vi "CRC16-接收校验.vi"(0 "读取缓冲区":string) -> (1 "净数据":string, 2 "CRC？":bool)   [LabVIEW 2017]
doc: "CRC16校验，输入待校验十六进制字符串，输出CRC校验码十六进制字符串高低位。"
panel:
  out "CRC16":string
  out "CRCL":string
  out "CRCH":string
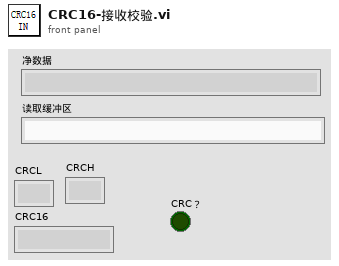
[diagram p1: front panel]
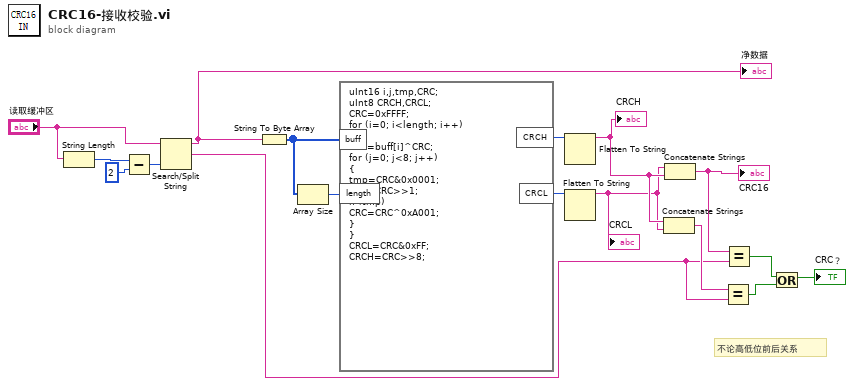
[diagram p0: block diagram]
diagram:
  # "不论高低位前后关系"
  n1 = String Length(string="读取缓冲区") -> (length=w11:i32)
  n2 = Subtract(x=w11, y=2) -> (x-y=w13:i32)
  n3 = Search/Split String(string="读取缓冲区", offset (0)=w13) -> (substring before match=w10:string, match + rest of string=w3:string)  [unwired: 1 in, 1 out]
  "净数据" <- w10
  n4 = String To Byte Array(string=w10) -> (unsigned byte array=w17:u8[])
  n5 = Array Size(array=w17) -> (size(s)=w16:i32)
  n6 = formula code="uInt16 i,j,tmp,CRC;\nuInt8 CRCH,CRCL;\nCRC=0xFFFF;\nfor (i=0; i<length; i++)\n{\nCRC=buff[i]^CRC;\nfor (j=0; j<8; j++)\n{\ntmp=CRC&0x0001;\nCRC=CRC>>1;\nif (tmp) \nCRC=CRC^0xA001;\n}\n}\nCRCL=CRC&0xFF;\nCRCH=CRC>>8;"("buff"=w17, "length"=w16) -> ("CRCH"=w15:u8, "CRCL"=w14:u8)
  n7 = Flatten To String(anything=w15) -> (data string=w6:string)  [unwired: 3 in, 2 out]
  "CRCH" <- w6
  n8 = Flatten To String(anything=w14) -> (data string=w5:string)  [unwired: 3 in, 2 out]
  "CRCL" <- w5
  n9 = Concatenate Strings(w6, w5) -> (w4:string)
  n10 = Concatenate Strings(w5, w6) -> (w9:string)
  "CRC16" <- w9
  n11 = Equal?(x=w4, y=w3) -> (x = y?=w1:bool)
  n12 = Equal?(x=w9, y=w3) -> (x = y?=w7:bool)
  n13 = Or(x=w7, y=w1) -> (x .or. y?=→"CRC？":bool)
